vi "Labview script.vi"() -> ()   [LabVIEW 2022 SP3]
uses:
  <vilib>/Analysis/3filter.llb/Filter Passband Type.ctl
  <vilib>/DAQmx/read.llb/DAQmx Read (Analog 1D DBL 1Chan NSamp).vi
  <vilib>/DAQmx/create/channels.llb/DAQmx Create Channel (AI-Voltage-Basic).vi
  <vilib>/DAQmx/configure/timing.llb/DAQmx Timing (Sample Clock).vi
  <vilib>/DAQmx/miscellaneous.llb/DAQmx Fill In Error Info.vi
  <vilib>/Analysis/3filter.llb/Butterworth Filter (DBL).vi
  <vilib>/Analysis/NI_AALBase.lvlib
  <vilib>/Analysis/NI_AAL_SigProc.lvlib
  <vilib>/Analysis/NI_AALPro.lvlib
panel:
  in  "Sorting Threshold low":dbl=100.0 format="%0.2f"
  in  "Time (s)":dbl=15.0 caption="Time Target (s)"
  out "Total Droplets\nin Histogram":dbl
  out "Droplets Outside Histogram":cluster{"total":i32, "below":i32, "above":i32}
  out "Percentage":dbl
  out "Sorted Droplets":i32
  in  "Sorting Threshold up":dbl=100.0 format="%0.2f"
  out "Raw Signal":cluster{dbl[], "data":dbl[]}(graph)
  out "Time Vector":dbl[](array[numeric])
  out "Filtered Signal":cluster{dbl[], "Filtered X":dbl[]}[](graph)
  in  "Save Filtered Data":bool
  in  "Path and Filename 2":path=path "C:/Users/Administrator/Documents/Philip/Data/filtered.txt" caption="Filename"
  out "Droplet Frequency":dbl
  in  "Path and Filename 3":path=path "C:/Users/Administrator/Documents/Philip/Data/test.txt" caption="Filename"
  in  "Save Histogram":bool
  in  "Add":bool
  in  "Start/Reset":bool
  out "Current Histogram":T1(graph)
  in  "Bins":i32=1000
  in  "Min":dbl format="%0.2f"
  in  "Max":dbl=400.0 format="%0.2f"
  out "Amplitudes":dbl[](array[numeric])
  out "Power Spectrum":T2(graph)
  in  "Peak Depth":dbl=50.0 format="%0.2f"
  in  "Peak width":i32=10 min=3
  in  "Filter on":bool=TRUE
  out "Time Span (ms)":dbl
  in  "Number of Samples":i32=1000
  in  "Order":i32=2
  in  "Cutoff Frequency (Hz)":dbl(slide)=16768.32936811008 scale=1.0..1000000.0
  out "Time Resolution (us)":dbl
  out "Clock Frequency":dbl
  in  "Unit":dbl(ring)=1000.0 items=["Hz"=1.0, "kHz"=1000.0]
  in  "Select Clock Frequency":dbl=50.0 format="%#.6g"
  in  "Path and Filename":path=path "C:/Users/Administrator/Documents/Philip/Data/test.txt" caption="Filename"
  in  "Save Raw Data":bool
  in  "stop":bool
  out "Cumulative Histogram":T1(graph)
  # "Aquisition Settings"
  # "Filter Settings"
  # "Peak Detection Settings"
  # "Histogram Settings"
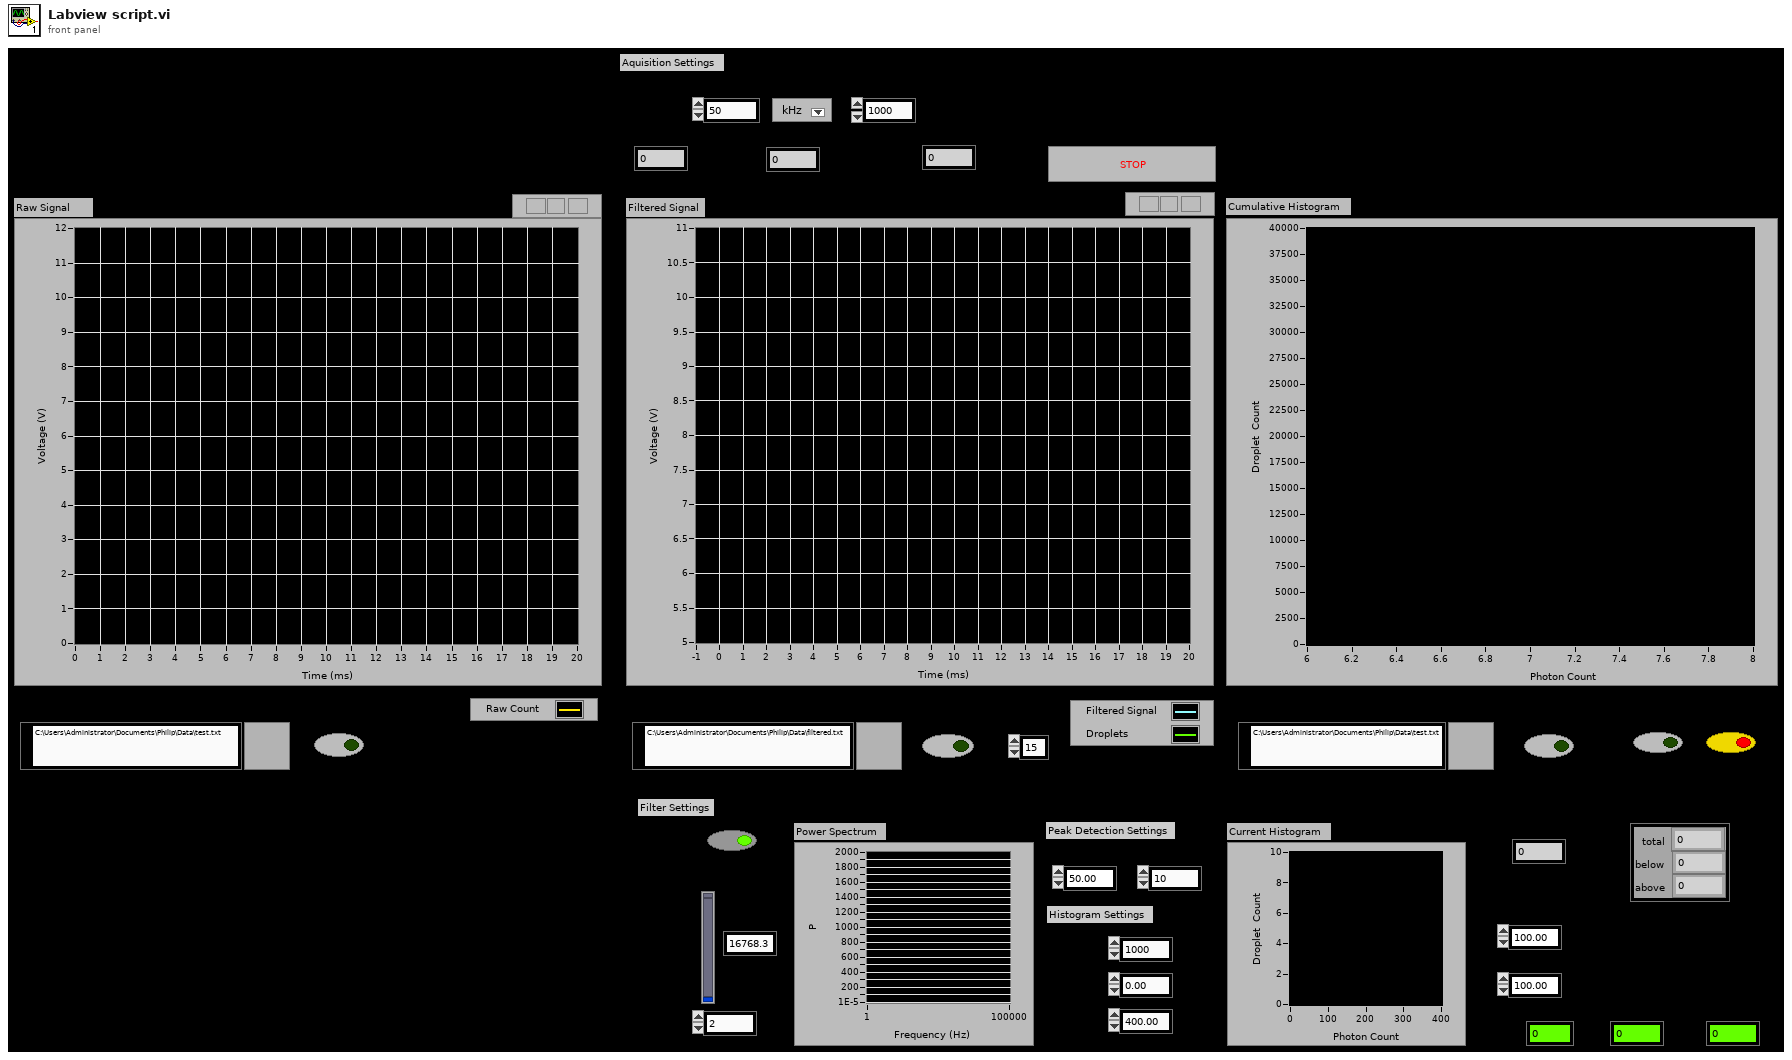
[diagram p1: front panel]
types:
  T1 = cluster{"X Values":dbl[], "Histogram: h(x)":i32[]}
  T2 = cluster{dbl[], "Power Spectrum (V^2 rms)":dbl[]}[]
  T3 = typedef "NI_AALBase.lvlib/Filter Passband Type.ctl" = enum32{"Lowpass", "Highpass", "Bandpass", "Bandstop"}
  T4 = cluster{"Time Vector":dbl[], "Amplitudes":dbl[]}[]
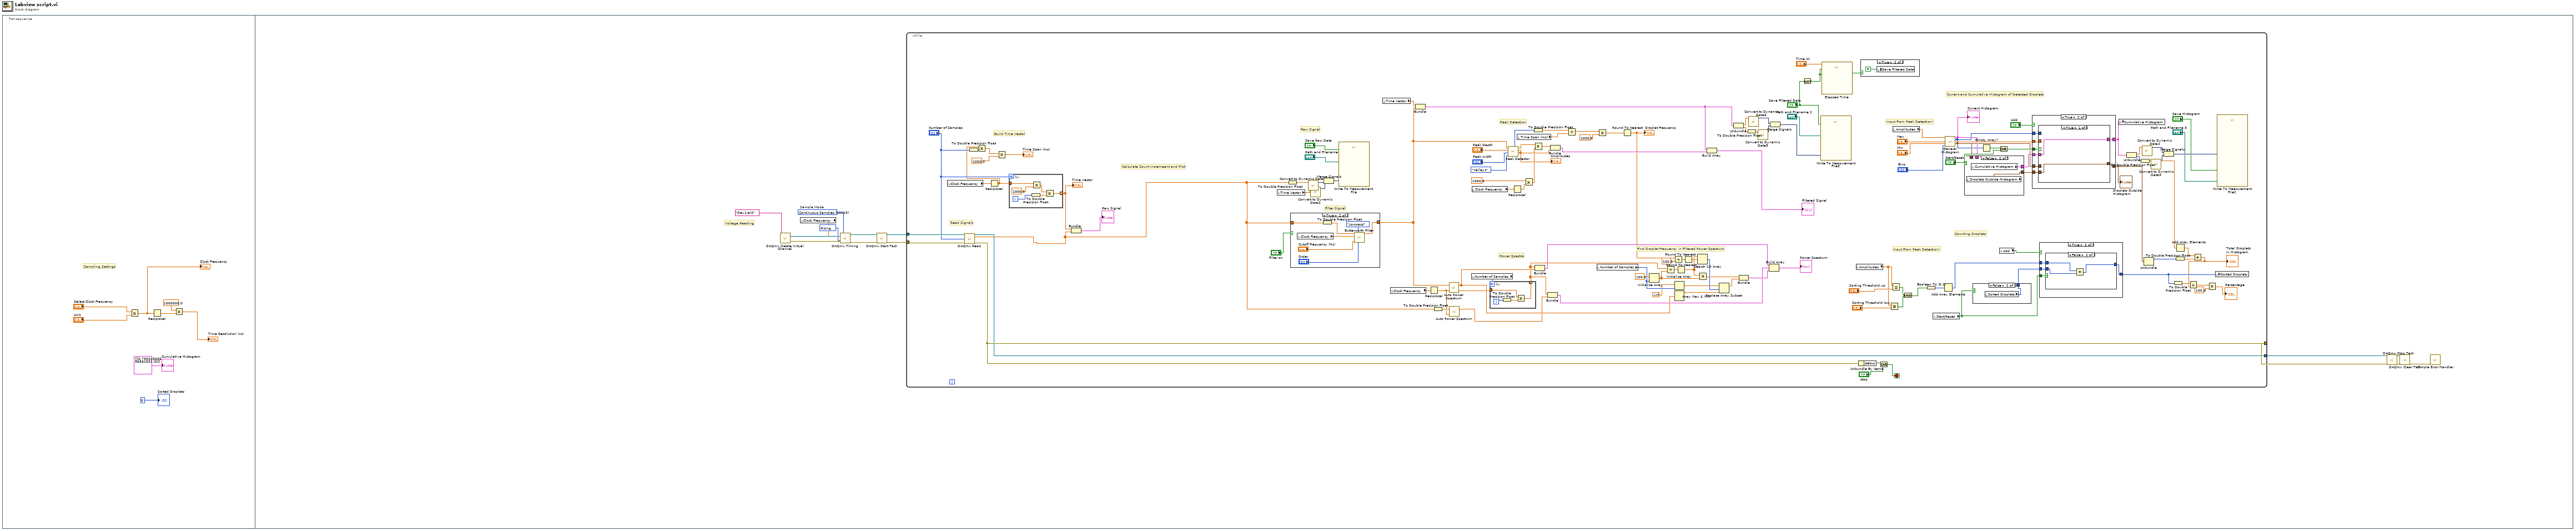
[diagram p0: block diagram]
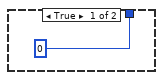
[diagram p5: hidden frame]
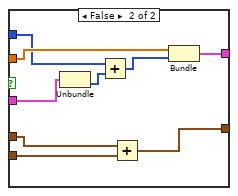
[diagram p7: hidden frame]
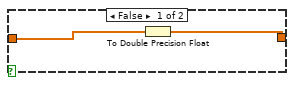
[diagram p9: hidden frame]
diagram:
  n1 = flat-sequence {
    frame #0 {
      # "Sampling Settings"
      n2 = Multiply(x="Select Clock Frequency", y="Unit") -> (x*y=w4:dbl)
      "Clock Frequency" <- w4
      n3 = Reciprocal(x=w4) -> (1/x=w3:dbl)
      n4 = Multiply(x=1000000.0, y=w3) -> (x*y=→"Time Resolution (us)":dbl)
      "Cumulative Histogram" <- T1 {"X Values"=[0.7300436369656153], "Histogram: h(x)"=[0]} ("Cumulative Histogram")
      "Sorted Droplets" <- 0 ("Sorted Droplets")
    }
    frame #1 {
      w16 = 10280 items=["Rising"=10280, "Falling"=10171] ("active edge")
      w13 = 10123 items=["Finite Samples"=10178, "Continuous Samples"=10123, "Hardware Timed Single Point"=12522]  # Sample Mode
      # "Voltage Reading"
      n5 = call-poly <vilib>:"DAQmx Create Virtual Channel.vi"("physical channels"=tag "Dev1/ai0") -> ("task out"=w15:refnum<k21>, "error out"=w18:errorcluster)  [unwired: 13 in]
      n6 = local read "Clock Frequency"() -> (w14:dbl)
      n7 = call-poly <vilib>:"DAQmx Timing.vi"("task/channels in"=w15, "sample mode"=w13, "rate"=w14, "active edge"=w16, "error in"=w18) -> ("task out"=w12:refnum<k21>, "error out"=w10:errorcluster)  [unwired: 9 in]
      n8 = call <vilib>:"DAQmx Start Task.vi"("task/channels in"=w12, "error in"=w10) -> ("task out"=w11:refnum<k21>, "error out"=w9:errorcluster)  [unwired: 12 in]
      n9 = while {
        tunnel: [w37] -> w23
        tunnel: w11 -> [w72]
        tunnel: [w66] -> w21
        tunnel: w9 -> [w38]
        stop <- w149 stop-if-true
        # "Calculate Count Incremeent and Plot"
        # "Read Signals"
        # "Build Time Vector"
        # "Input From Peak Detection!"
        # "Counting Droplets"
        # "Input From Peak Detection!"
        # "Current and Cumulative Histogram of Detected Droplets"
        # "Find Droplet Frequency in Filtered Power Spectrum"
        # "Power Spectra"
        # "Raw Signal"
        # "Peak Detection"
        # "Filter Signal"
        n10 = local read "Clock Frequency"() -> (w51:dbl)
        n11 = call-poly <vilib>:"DAQmx Read.vi"("task/channels in"=w72, "number of samples per channel"="Number of Samples", "error in"=w38) -> ("task out"=w66:refnum<k21>, "data"=w29:dbl[], "error out"=w37:errorcluster)  [unwired: 10 in]
        n12 = To Double Precision Float(number="Number of Samples") -> (double precision float=w50:dbl)
        n13 = Reciprocal(x=w51) -> (1/x=w49:dbl)
        n14 = Multiply(x=w49, y=w50) -> (x*y=w48:dbl)
        n15 = Multiply(x=w48, y=1000.0) -> (x*y=→"Time Span (ms)":dbl)
        n16 = for {
          N: "Number of Samples" -> [_]
          tunnel: [w157] -> w67 mode=indexing
          tunnel: w49 -> [w156]
          i -> [w158]
          n17 = To Double Precision Float(number=w158) -> (double precision float=w155:dbl)
          n18 = Multiply(x=w156, y=1000.0) -> (x*y=w154:dbl)
          n19 = Multiply(x=w154, y=w155) -> (x*y=w157:dbl)
        }
        "Time Vector" <- w67
        n20 = Bundle(w67, "data"=w29) -> (→"Raw Signal":cluster{dbl[], "data":dbl[]})  [unwired: 1 in]
        n21 = local read "Time Vector"() -> (w65:dbl[])
        n22 = To Double Precision Float(number=w29) -> (double precision float=w147:dbl[])
        n23 = case shown="True" "Filter on" {
          tunnel: w29 -> [w200 w207]
          tunnel: [w199 w203] -> w71
          frame False {
            n24 = To Double Precision Float(number=w200) -> (double precision float=w199:dbl[])
          }
          frame True {
            n25 = local read "Clock Frequency"() -> (w205:dbl)
            n26 = To Double Precision Float(number=w207) -> (double precision float=w206:dbl[])
            n27 = call-poly <vilib>:"Butterworth Filter.vi"("order"="Order", "filter type"=Filter_Passband_Type."Lowpass", "low cutoff freq: fl"="Cutoff Frequency (Hz)", "sampling freq: fs"=w205, "X"=w206) -> ("Filtered X"=w203:dbl[])  [unwired: 3 in, 1 out]
          }
        }
        n28 = call "Convert to Dynamic Data"("Array"=w147) -> ("Dynamic Data Type"=w148:dynamicdata)  [unwired: 3 in]
        n29 = call "Convert to Dynamic Data2"("Array"=w65) -> ("Dynamic Data Type"=w95:dynamicdata)  [unwired: 3 in]
        n30 = Merge Signals(w95, w148) -> (w96:dynamicdata)
        n31 = call "Write To Measurement File"("Signals"=w96, "Enable"="Save Raw Data", "Filename"="Path and Filename") -> ()  [unwired: 14 in, 3 out]
        n32 = local read "Time Vector"() -> (w64:dbl[])
        n33 = local read "Clock Frequency"() -> (w127:dbl)
        n34 = Bundle("Time Vector"=w64, "Filtered X"=w71) -> (w70:cluster{"Time Vector":dbl[], "Filtered X":dbl[]})  [unwired: 1 in]
        n35 = Reciprocal(x=w127) -> (1/x=w73:dbl)
        n36 = To Double Precision Float(number=w29) -> (double precision float=w78:dbl[])
        n37 = call <vilib>:"Auto Power Spectrum.vi"("dt"=w73, "Signal (V)"=w71) -> ("df"=w129:dbl, "Power Spectrum (V^2 rms)"=w87:dbl[])
        n38 = call <vilib>:"Auto Power Spectrum.vi"("dt"=w73, "Signal (V)"=w78) -> ("Power Spectrum (V^2 rms)"=w77:dbl[])  [unwired: 1 out]
        n39 = local read "Number of Samples"() -> (w117:i32)
        n40 = local read "Clock Frequency"() -> (w138:dbl)
        n41 = for {
          N: w117 -> [_]
          tunnel: w129 -> [w195]
          tunnel: [w196] -> w76 mode=indexing
          i -> [w198]
          n42 = To Double Precision Float(number=w198) -> (double precision float=w197:dbl)
          n43 = Multiply(x=w195, y=w197) -> (x*y=w196:dbl)
        }
        n44 = call <vilib>:"Peak Detector.vi"("peaks/valleys"=enum32{"Peaks", "Valleys"}."Valleys", "width"="Peak width", "threshold"="Peak Depth", "X"=w71) -> ("Amplitudes"=w140:dbl[], "Locations"=w133:dbl[], "# found"=w132:i32)  [unwired: 3 in, 2 out]
        "Amplitudes" <- w140
        n45 = Reciprocal(x=w138) -> (1/x=w137:dbl)
        n46 = local read "Time Span (ms)"() -> (w130:dbl)
        n47 = Multiply(x=1000.0, y=w137) -> (x*y=w134:dbl)
        n48 = To Double Precision Float(number=w132) -> (double precision float=w131:dbl)
        n49 = Multiply(x=w133, y=w134) -> (x*y=w139:dbl[])
        n50 = Bundle(w76, "Power Spectrum (V^2 rms)"=w87) -> (w128:cluster{dbl[], "Power Spectrum (V^2 rms)":dbl[]})  [unwired: 1 in]
        n51 = Bundle(w76, "Power Spectrum (V^2 rms)"=w77) -> (w74:cluster{dbl[], "Power Spectrum (V^2 rms)":dbl[]})  [unwired: 1 in]
        n52 = Bundle(w139, "Amplitudes"=w140) -> (w135:cluster{dbl[], "Amplitudes":dbl[]})  [unwired: 1 in]
        n53 = Divide(x=w131, y=w130) -> (x/y=w126:dbl)
        n54 = local read "Number of Samples"() -> (w109:i32)
        n55 = Multiply(x=w126, y=1000.0) -> (x*y=w114:dbl)
        n56 = Round To Nearest(number=w114) -> (nearest integer value=w122:dbl)
        "Droplet Frequency" <- w122
        n57 = Initialize Array(100.0 ("element"), w109) -> (w111:dbl[])
        n58 = Divide(x=w76, y=w111) -> (x/y=w119:dbl[])
        n59 = Divide(x=w122, y=100.0) -> (x/y=w116:dbl)
        n60 = Initialize Array(-inf, w109) -> (w123:dbl[])
        n61 = Array Max & Min(array=w87) -> (max value=w108:dbl)  [unwired: 3 out]
        n62 = Round To Nearest(number=w119) -> (nearest integer value=w120:dbl[])
        n63 = Round To Nearest(number=w116) -> (nearest integer value=w113:dbl)
        n64 = Search 1D Array(1D array=w120, element=w113) -> (index of element=w124:i32)  [unwired: 1 in]
        n65 = Multiply(x=w120, y=w111) -> (x*y=w112:dbl[])
        n66 = Build Array(w70, w135) -> (→"Filtered Signal":T4)
        n67 = Replace Array Subset(array=w123, new element=w108, index=w124) -> (w121:dbl[])
        n68 = Unbundle(w70) -> ("Time Vector"=w83:dbl[], "Filtered X"=w81:dbl[])
        n69 = Bundle(w112, w121) -> (w75:cluster{dbl[], dbl[]})  [unwired: 1 in]
        n70 = To Double Precision Float(number=w81) -> (double precision float=w85:dbl[])
        n71 = call "Convert to Dynamic Data6"("Array"=w83) -> ("Dynamic Data Type"=w84:dynamicdata)  [unwired: 3 in]
        n72 = call "Convert to Dynamic Data5"("Array"=w85) -> ("Dynamic Data Type"=w82:dynamicdata)  [unwired: 3 in]
        n73 = Build Array(w128, w74, w75) -> (→"Power Spectrum":T2)
        n74 = Merge Signals(w84, w82) -> (w80:dynamicdata)
        n75 = Not(x="Save Filtered Data") -> (.not. x?=w33:bool)
        n76 = call "Write To Measurement File3"("Signals"=w80, "Enable"="Save Filtered Data", "Filename"="Path and Filename 2") -> ()  [unwired: 14 in, 3 out]
        n77 = call "Elapsed Time"("Time Target (s)"="Time (s)", "Reset"=w33, "Auto Reset"=w33) -> ("Time has Elapsed"=w34:bool)  [unwired: 9 in, 7 out]
        n78 = local read "Amplitudes"() -> (w28:dbl[])
        n79 = Unbundle By Name(w37) -> ("status"=w150:bool)
        n80 = case shown="True" w34 {
          frame False {
          }
          frame True {
            n81 = local write "Save Filtered Data"(FALSE ("Save Filtered Data")) -> ()
          }
        }
        n82 = Or(x=w150, y="stop") -> (x .or. y?=w149:bool)
        n83 = Greater Or Equal?(x=w28, y="Sorting Threshold low") -> (x >= y?=w26:bool[])
        n84 = Less Or Equal?(x=w28, y="Sorting Threshold up") -> (x <= y?=w25:bool[])
        n85 = local read "Amplitudes"() -> (w107:dbl[])
        n86 = And(x=w25, y=w26) -> (x .and. y?=w24:bool[])
        n87 = Boolean To (0,1)(Boolean=w24) -> (0, 1=w62:i16[])
        n88 = local read "Start/Reset"() -> (w52:bool)
        n89 = Add Array Elements(numeric array=w62) -> (sum=w60:i16)
        n90 = call <vilib>:"General Histogram.vi"("X"=w107, "max"="Max", "min"="Min", "# bins"="Bins") -> ("Histogram Graph"=w32:T1, "Histogram"=w101:i32[], "Axis"=w103:dbl[], "# outside"=w31:cluster{"total":i32, "below":i32, "above":i32})  [unwired: 7 in, 1 out]
        "Current Histogram" <- w32
        n91 = case shown="False" "Start/Reset" {
          tunnel: [w192 w194] -> w102
          tunnel: w32 -> [w192 _]
          tunnel: w31 -> [w191 _]
          tunnel: [w191 w193] -> w30
          frame True {
          }
          frame False {
            n92 = local read "Droplets Outside Histogram"() -> (w193:cluster{"total":i32, "below":i32, "above":i32})
            n93 = local read "Cumulative Histogram"() -> (w194:T1)
          }
        }
        n94 = case shown="False" w52 {
          tunnel: [0 w169] -> w63
          frame True {
          }
          frame False {
            n95 = local read "Sorted Droplets"() -> (w169:i32)
          }
        }
        n96 = Empty Array?(array=w101) -> (empty?=w98:bool)
        n97 = Or(x=w98, y="Start/Reset") -> (x .or. y?=w99:bool)
        n98 = local read "Add"() -> (w53:bool)
        n99 = case shown="True" "Add" {
          tunnel: w103 -> [_ w179]
          tunnel: w102 -> [w171 w178]
          tunnel: w101 -> [_ w177]
          tunnel: w99 -> [_ w176]
          tunnel: [w171 w175] -> w94
          tunnel: w30 -> [_ w174]
          tunnel: w31 -> [w170 w173]
          tunnel: [w170 w172] -> w42
          frame False {
          }
          frame True {
            n100 = case shown="True" w176 {
              tunnel: w179 -> [_ w188]
              tunnel: w177 -> [_ w187]
              tunnel: [w181 w186] -> w175
              tunnel: w178 -> [w181 w185]
              tunnel: w174 -> [w180 w183]
              tunnel: w173 -> [_ w182]
              tunnel: [w180 w184] -> w172
              frame True {
              }
              frame False {
                n101 = Unbundle(w185) -> ("Histogram: h(x)"=w190:i32[])  [unwired: 1 out]
                n102 = Add(x=w187, y=w190) -> (x+y=w189:i32[])
                n103 = Add(x=w182, y=w183) -> (x+y=w184:cluster{"total":i32, "below":i32, "above":i32})
                n104 = Bundle("Axis"=w188, w189) -> (w186:cluster{"Axis":dbl[], i32[]})  [unwired: 1 in]
              }
            }
          }
        }
        "Droplets Outside Histogram" <- w42
        n105 = case shown="True" w53 {
          tunnel: w52 -> [_ w163]
          tunnel: [w159 w161] -> w57
          tunnel: w63 -> [w159 w162]
          tunnel: w60 -> [_ w160]
          frame False {
          }
          frame True {
            n106 = case shown="False" w163 {
              tunnel: w162 -> [w164 w167]
              tunnel: [w164 w166] -> w161
              tunnel: w160 -> [_ w165]
              frame True {
              }
              frame False {
                n107 = Add(x=w165, y=w167) -> (x+y=w166:i32)
              }
            }
          }
        }
        n108 = local write "Cumulative Histogram"(w94) -> ()
        n109 = Unbundle(w94) -> ("Axis"=w92:dbl[], "Histogram: h(x)"=w59:i32[])
        n110 = To Double Precision Float(number=w59) -> (double precision float=w58:dbl[])
        n111 = call "Convert to Dynamic Data4"("Array"=w92) -> ("Dynamic Data Type"=w90:dynamicdata)  [unwired: 3 in]
        n112 = Unbundle(w42) -> ("total"=w40:i32)  [unwired: 2 out]
        n113 = call "Convert to Dynamic Data3"("Array"=w58) -> ("Dynamic Data Type"=w93:dynamicdata)  [unwired: 3 in]
        n114 = Merge Signals(w90, w93) -> (w91:dynamicdata)
        n115 = To Double Precision Float(number=w57) -> (double precision float=w55:dbl)
        n116 = Add Array Elements(numeric array=w58) -> (sum=w56:dbl)
        n117 = To Double Precision Float(number=w40) -> (double precision float=w39:dbl)
        n118 = Add(x=w56, y=w39) -> (x+y=w41:dbl)
        "Total Droplets\nin Histogram" <- w41
        n119 = Divide(x=w55, y=w41) -> (x/y=w54:dbl)
        n120 = Multiply(x=w54, y=100.0) -> (x*y=→"Percentage":dbl)
        n121 = local write "Sorted Droplets"(w57) -> ()
        n122 = call "Write To Measurement File2"("Signals"=w91, "Enable"="Save Histogram", "Filename"="Path and Filename 3") -> ()  [unwired: 14 in, 3 out]
      }
      n123 = call <vilib>:"DAQmx Stop Task.vi"("task/channels in"=w21, "error in"=w23) -> ("task out"=w22:refnum<k21>, "error out"=w20:errorcluster)  [unwired: 12 in]
      n124 = call <vilib>:"DAQmx Clear Task.vi"("task in"=w22, "error in"=w20) -> ("error out"=w19:errorcluster)  [unwired: 13 in]
      n125 = call <vilib>:"Simple Error Handler.vi"("error in (no error)"=w19) -> ()  [unwired: 4 in, 5 out]
    }
  }
